vi "Tach_FPGA.vi"(6 "Analog In (Tach)":fxp<+/-,24,4> format="%.22g", 7 "Slope":enum16{"falling", "rising"}(ring), 9 "Threshold":fxp<+/-,16,16>, 11 "Hysteresis":fxp<+,1,0>=0.5 format="%.1g") -> (0 "Tach State":enum16{"Check Hysteresis", "Check Threshold"}(ring), 2 "Tach Period (uSec/pulse)":u32)   [LabVIEW 2012]
uses:
  Instance           1 17Saved   Tach_FPGA .vi
  <vilib>/rvi/Arithmetic/AddSubMult/XNode/nirviSatArithmetic.xnode
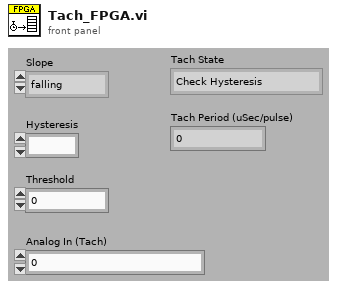
[diagram p1: front panel]
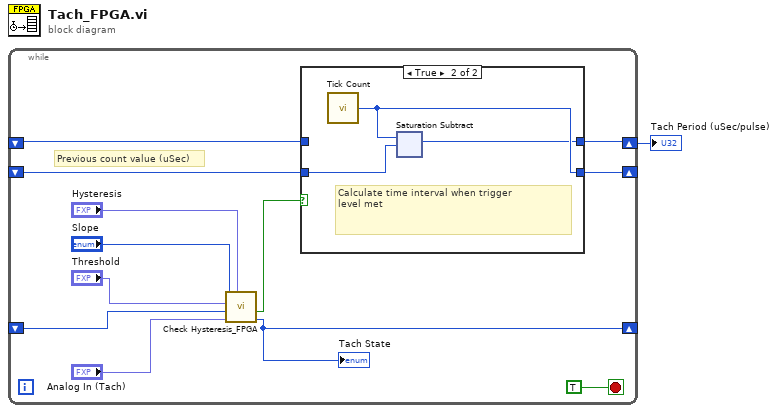
[diagram p0: block diagram]
diagram:
  n1 = while {
    shift-right: [w9] -> _
    shift-left: _ -> [w8]
    shift-right: [w7] -> _
    shift-left: _ -> [w6]
    shift-right: [w5] -> w1
    shift-left: _ -> [w4]
    stop <- TRUE stop-if-true
    # "Previous count value (uSec)"
    n2 = call "Check Hysteresis_FPGA.vi"("Hysteresis"="Hysteresis", "Analog In (Tach)"="Analog In (Tach)", "State In"=w6, "Threshold"="Threshold", "Slope"="Slope") -> ("State Out"=w7:enum16{"Check Hysteresis", "Check Threshold"}, "Event Ocurred?"=w13:bool)  [unwired: 2 in]
    "Tach State" <- w7
    n3 = case shown="True" w13 {
      tunnel: w8 -> [w15 w17]
      tunnel: [w15 w18] -> w9
      tunnel: [w14 w16] -> w5
      tunnel: w4 -> [w14 _]
      frame False {
      }
      frame True {
        # "Calculate time interval when trigger\nlevel met"
        n4 = call "Tick Count"() -> ("Tick Count(uSec)"=w18:u32)
        n5 = xnode ("Saturation Subtract")("x"=w18, "y"=w17) -> ("x-y"=w16:u32)
      }
    }
  }
  "Tach Period (uSec/pulse)" <- w1
